vi "get_cycle_properties.vi"(8 "error in (no error)":errorcluster, 11 "ScanModeTS090821Circular2D in":refnum<class "ImagingModeTS090821Circular2D.lvclass">) -> (0 "error out":errorcluster, 1 "number of cycles":i32, 2 "total number of pixels per cycle":i32, 3 "ScanModeTS090821Circular2D out":refnum<class "ImagingModeTS090821Circular2D.lvclass">, 4 "scan rate":dbl[unit], 5 "pixel frequency":dbl[unit], 7 "pixel dwell time":dbl[unit])   [LabVIEW 2010, in "ImagingModeTS090821Circular2D.lvclass"]
uses:
  ImagingModeTS090821Circular2D.lvclass
  ImagingModeTS090821Circular2D.lvclass/ImagingModeTS090821Circular2D.ctl
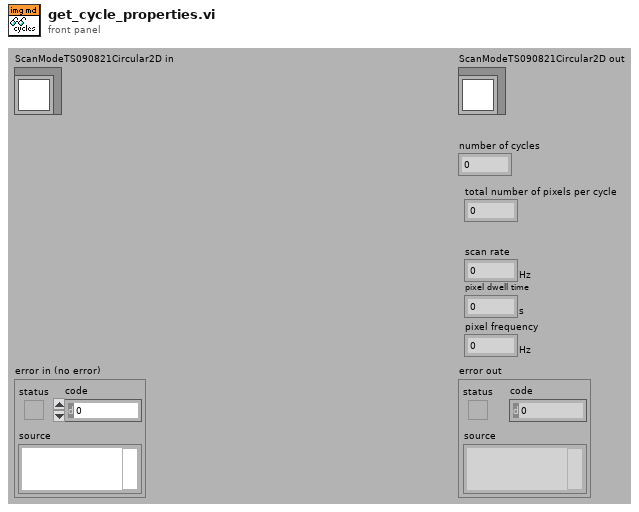
[diagram p1: front panel]
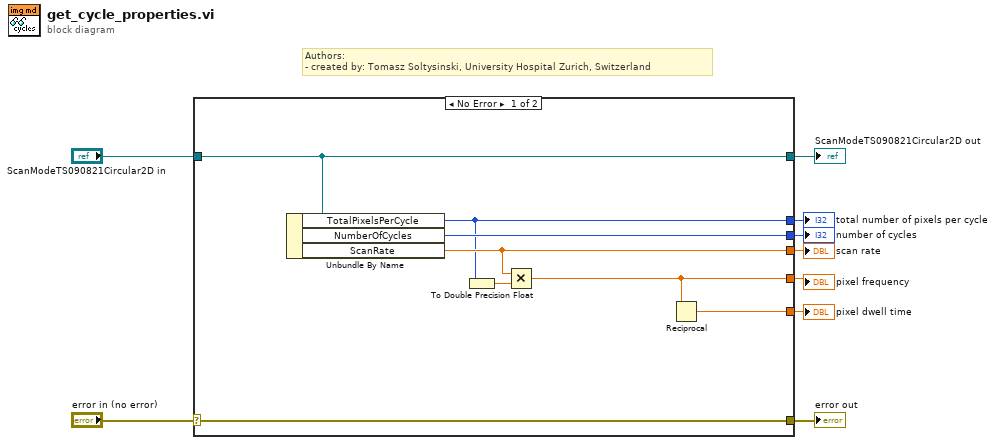
[diagram p0: block diagram]
diagram:
  # "Authors: \n- created by: Tomasz Soltysinski, University Hospital Zurich, Switzerland"
  n1 = case shown="No Error" "error in (no error)" {
    selector: "error in (no error)" -> [w17 w19]
    tunnel: [w17 w19] -> w8
    tunnel: [w16 w18] -> w6
    tunnel: "ScanModeTS090821Circular2D in" -> [w16 w18]
    tunnel: [w12 _] -> w5
    tunnel: [w15 _] -> w4
    tunnel: [w14 _] -> w3
    tunnel: [w10 _] -> w2
    tunnel: [w11 _] -> w1
    frame No Error {
      n2 = Unbundle By Name(w16) -> ("TotalPixelsPerCycle"=w12:i32, "NumberOfCycles"=w15:i32, "ScanRate"=w14:dbl[unit])
      n3 = To Double Precision Float(number=w12) -> (double precision float=w13:dbl)
      n4 = Multiply(x=w14, y=w13) -> (x*y=w11:dbl[unit])
      n5 = Reciprocal(x=w11) -> (1/x=w10:dbl[unit])
    }
    frame Error {
    }
  }
  "error out" <- w8
  "ScanModeTS090821Circular2D out" <- w6
  "total number of pixels per cycle" <- w5
  "number of cycles" <- w4
  "scan rate" <- w3
  "pixel dwell time" <- w2
  "pixel frequency" <- w1
